vi "QUIZ#1 (interfaz cmd AT).vi"() -> ()   [LabVIEW 2020]
panel:
  out "index of element":i32
  in  "nomtipo":string[](array[string])
  out "element":string
  out "index nombre":i32
  out "before substring":string
  out "es ? , sino sera =":string
  in  "Rpta":string[](array[string])
  in  "Numeric 4":i32
  in  "#args":string[](array[string])
  in  "Numeric 3":i32
  in  "Tipo":string[](array[string])
  in  "Numeric 2":i32
  in  "Nombre":string[](array[string])
  in  "Numeric":i32
  in  "Pulsador 3":bool
  in  "Pulsador 2":bool
  in  "Pulsador 1":bool
  out "Led 3":bool
  out "Led 2":bool
  out "Led 1":bool
  out "tiempo(ms)":i32=2000
  out "Contador":i32
  in  "Insertar trama":string
  out "RESPUESTA":string="\n      \n           "
  in  "Ingreso de comandos":string
  in  "?":bool
  # "DAVID GIRALDO VILLA.\nOSCAR ANDRES CORDOBA."
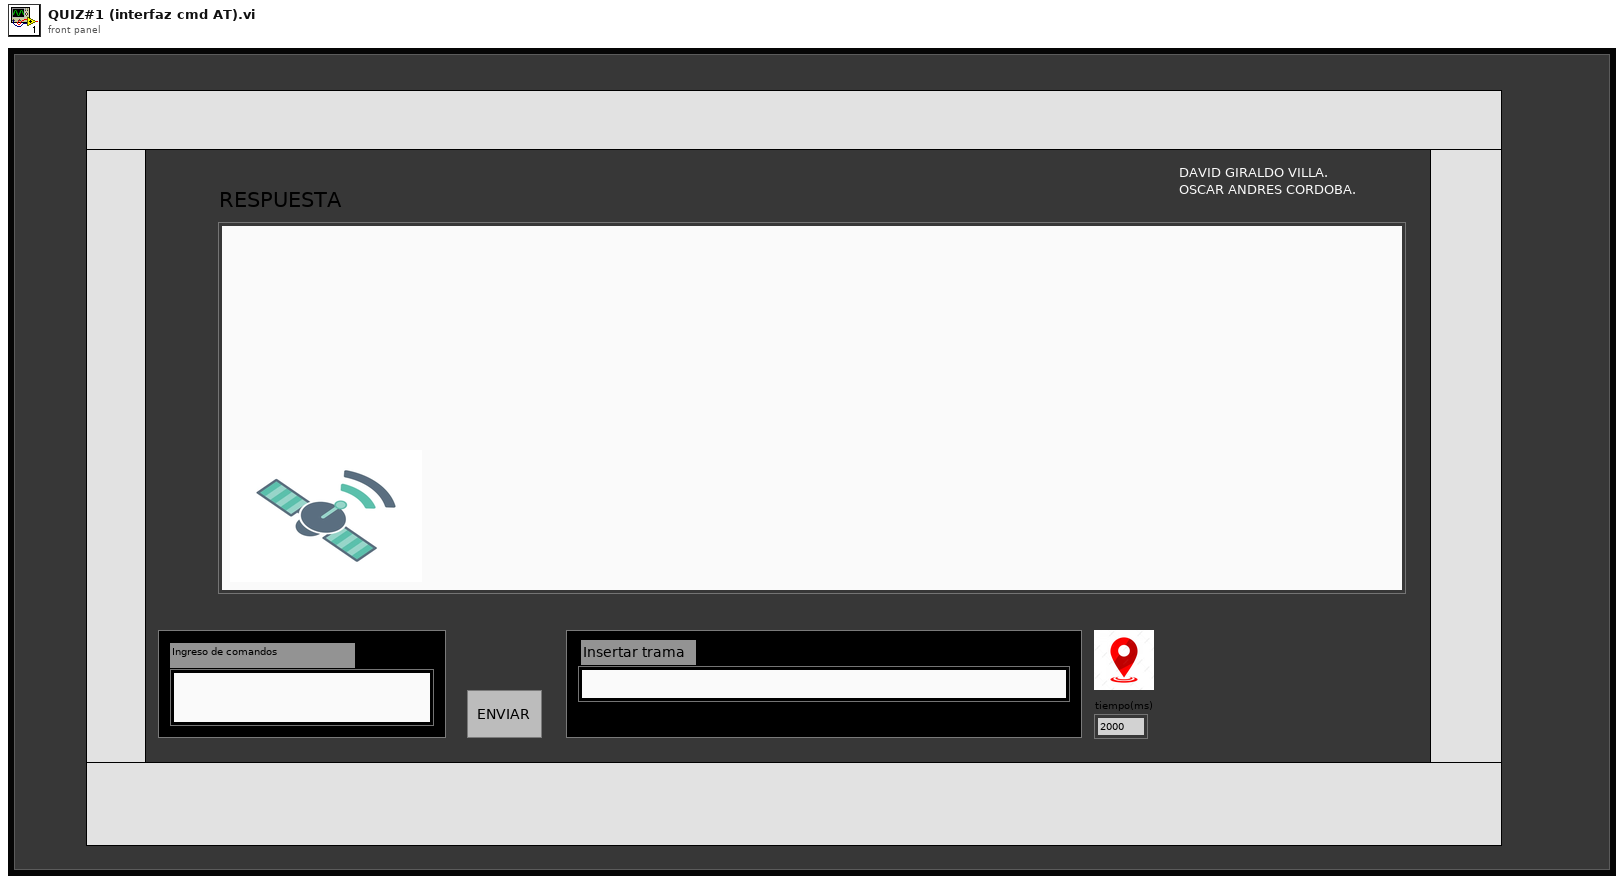
[diagram p1: front panel]
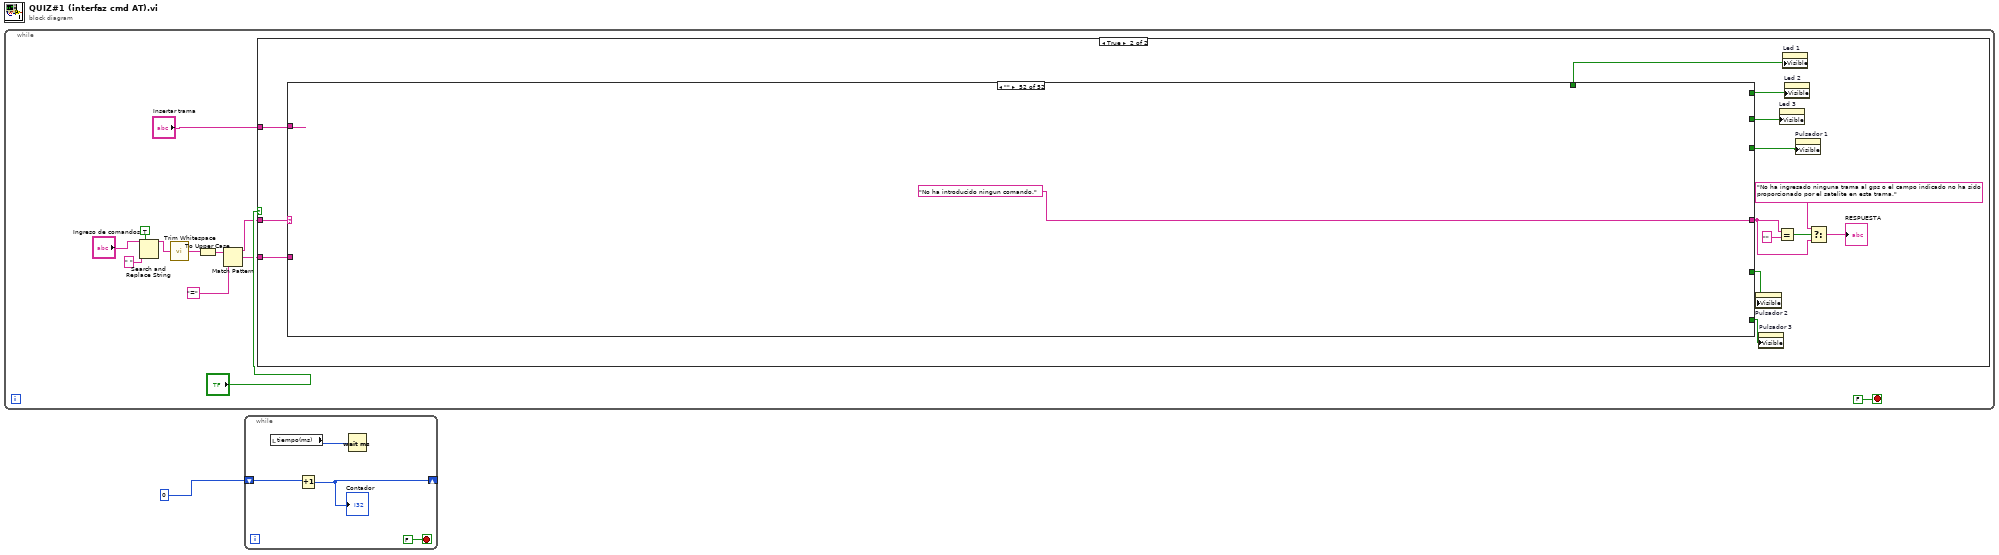
[diagram p0: block diagram]
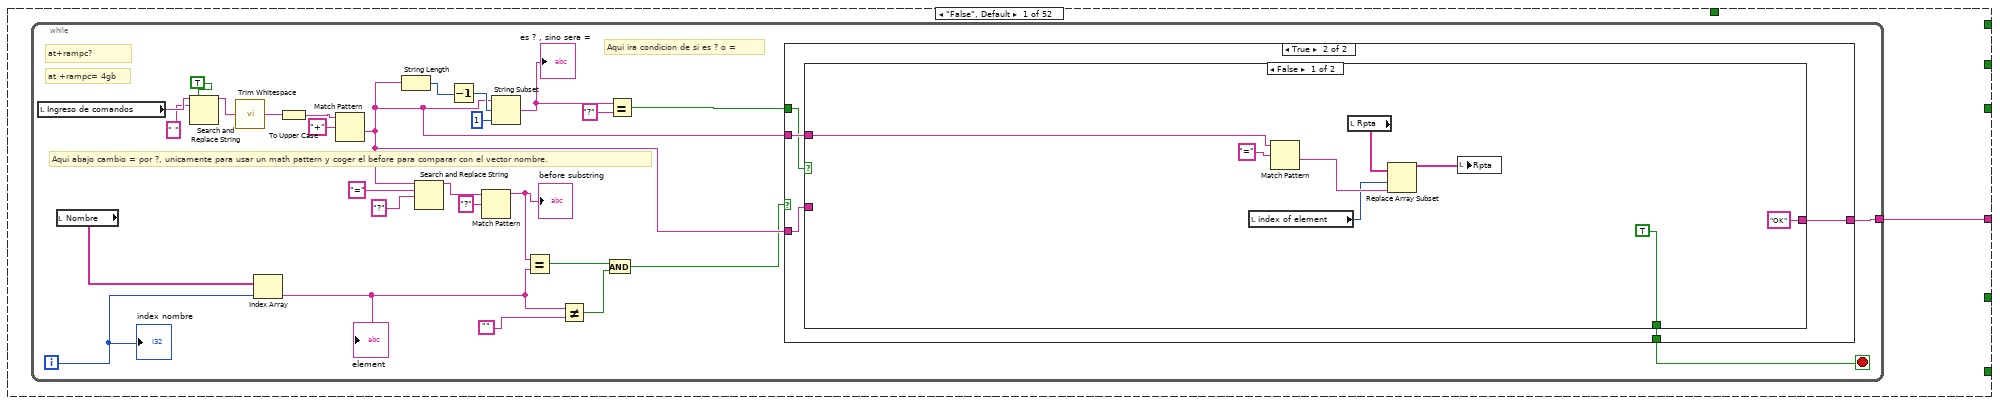
[diagram p3: hidden frame]
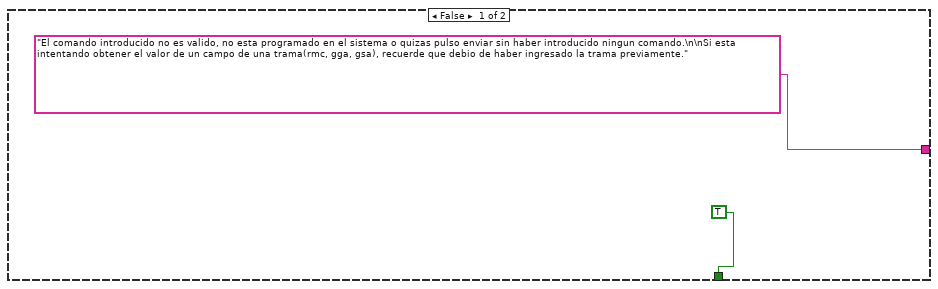
[diagram p4: hidden frame]
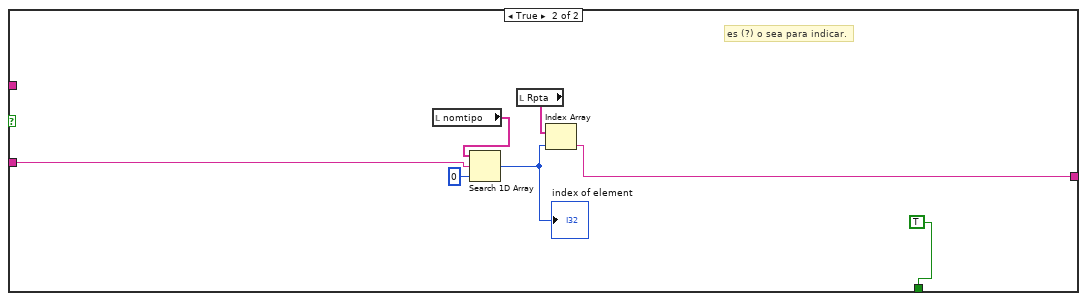
[diagram p5: hidden frame]
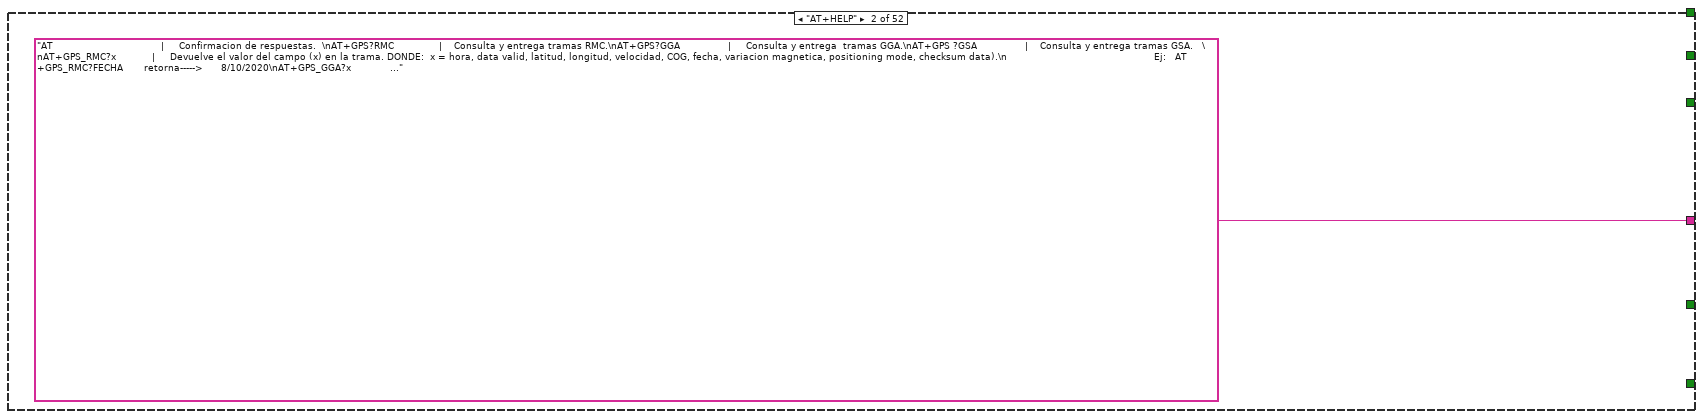
[diagram p6: hidden frame]
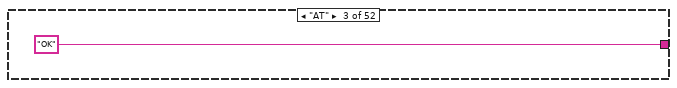
[diagram p7: hidden frame]
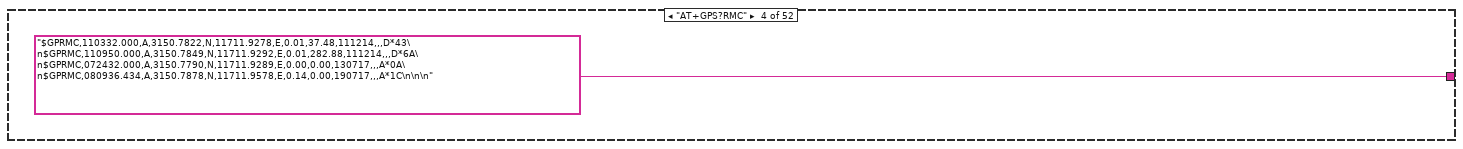
[diagram p8: hidden frame]
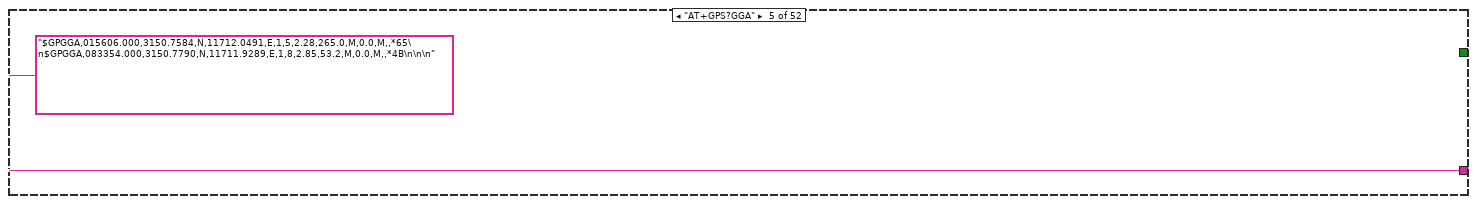
[diagram p9: hidden frame]
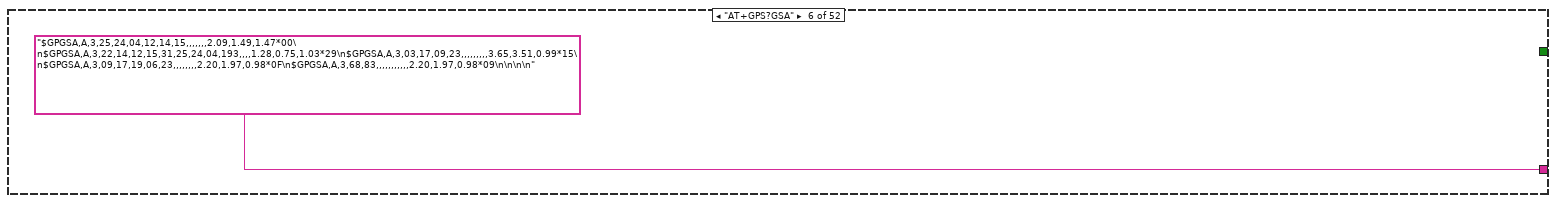
[diagram p10: hidden frame]
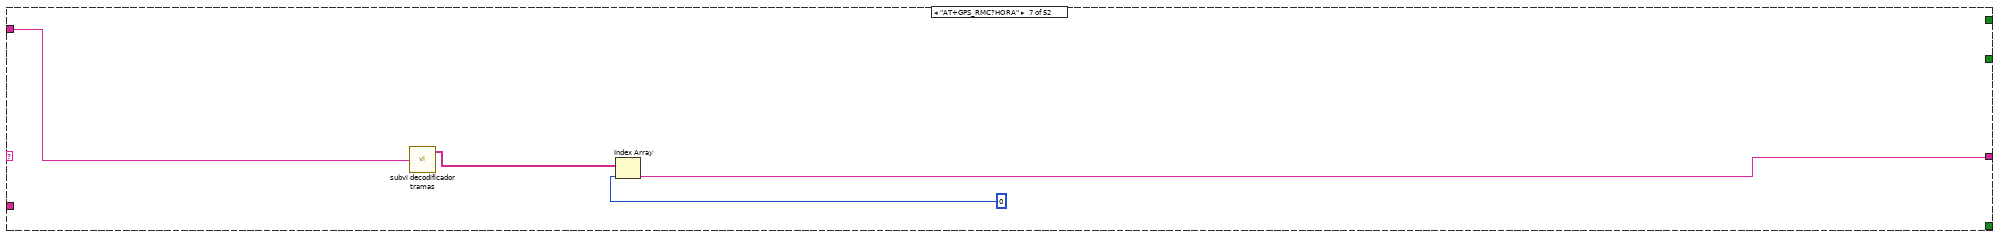
[diagram p11: hidden frame]
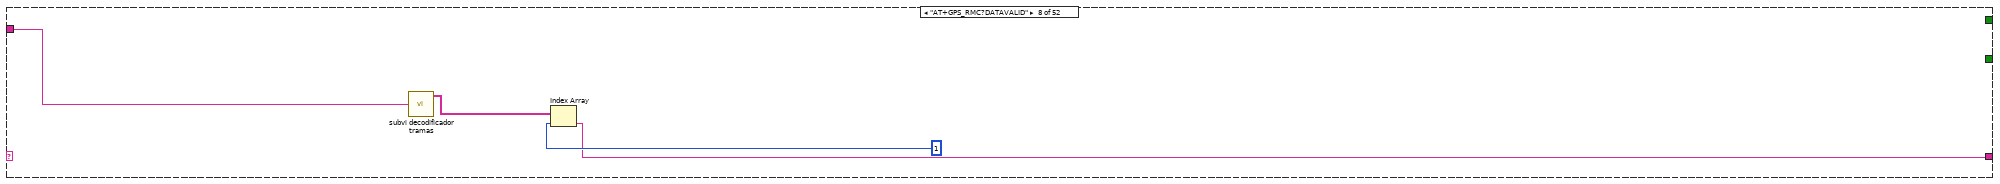
[diagram p12: hidden frame]
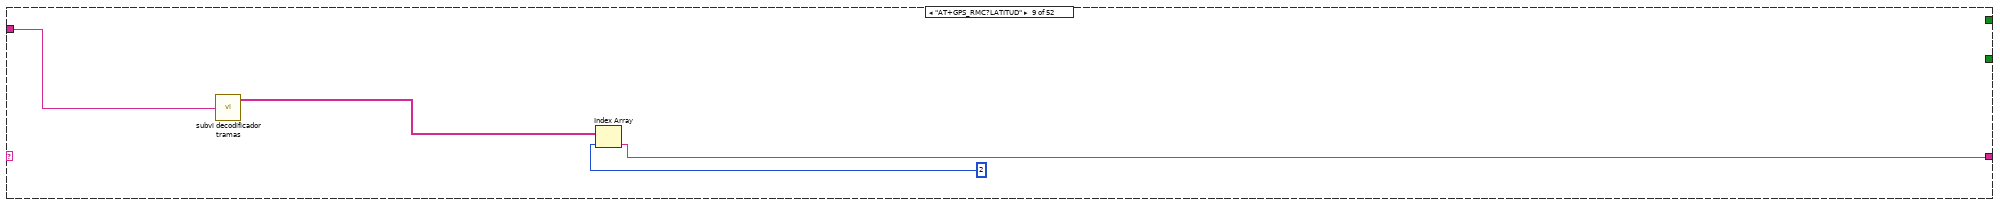
[diagram p13: hidden frame]
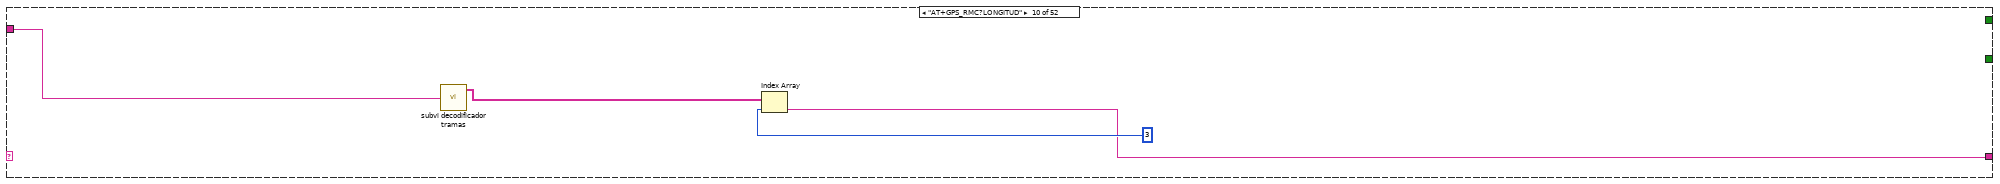
[diagram p14: hidden frame]
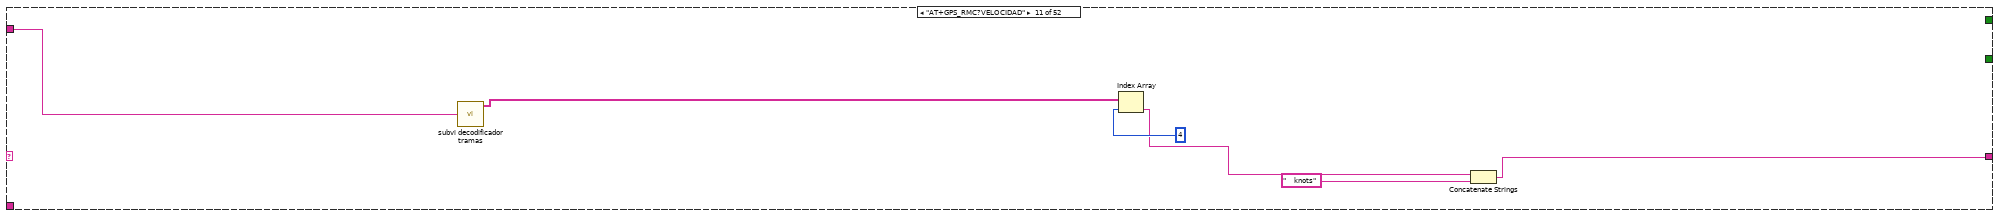
[diagram p15: hidden frame]
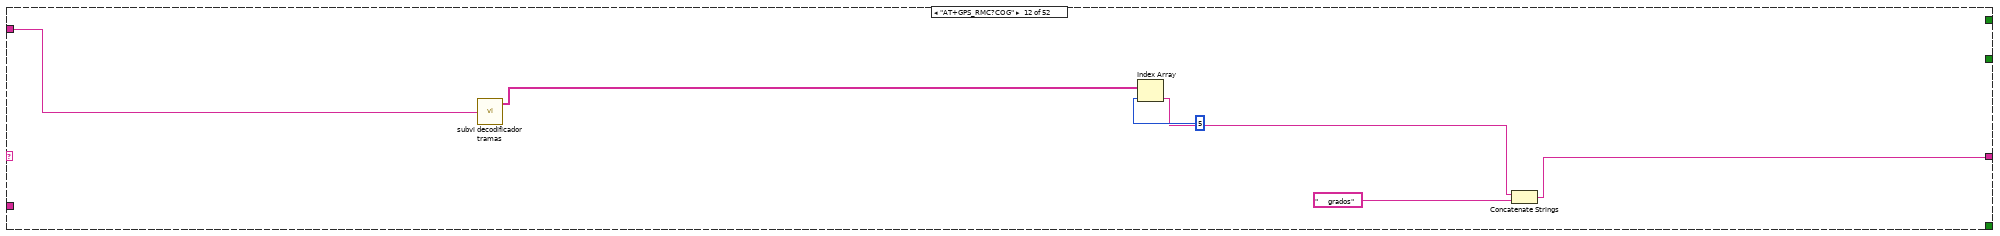
[diagram p16: hidden frame]
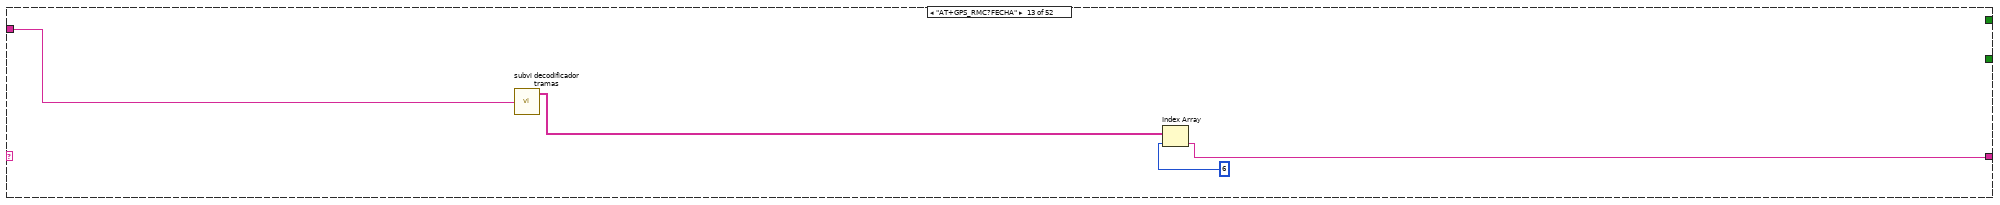
[diagram p17: hidden frame]
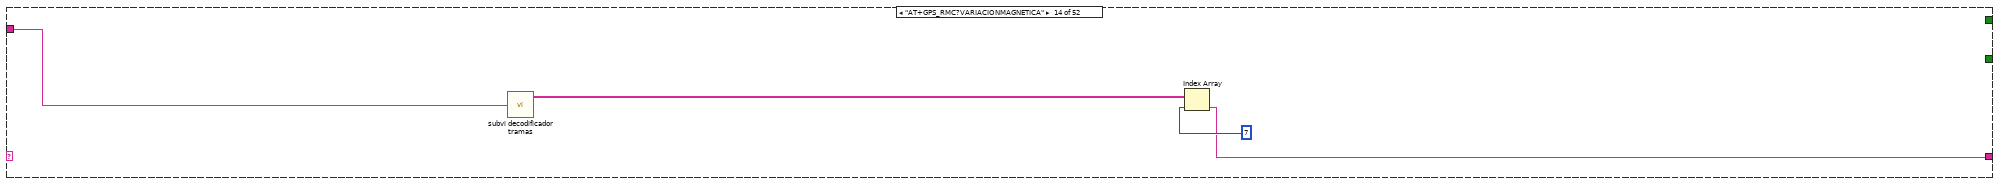
[diagram p18: hidden frame]
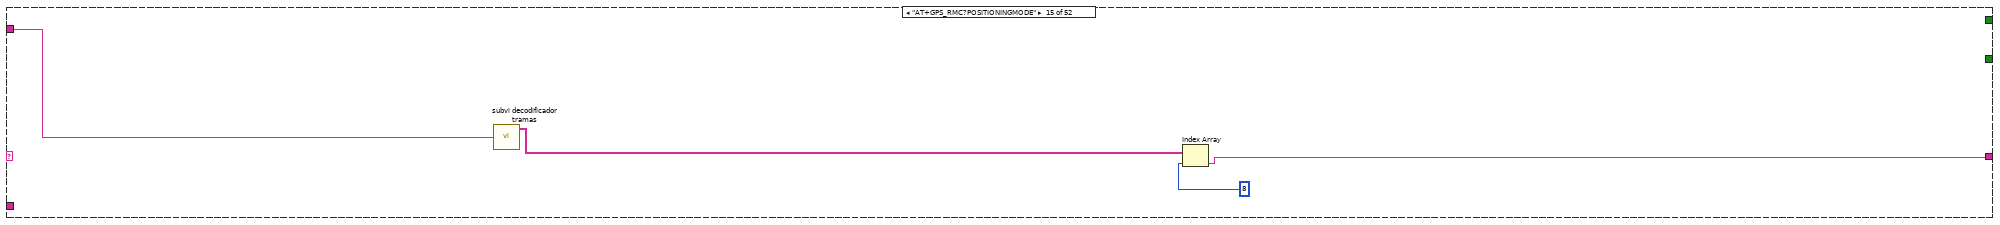
[diagram p19: hidden frame]
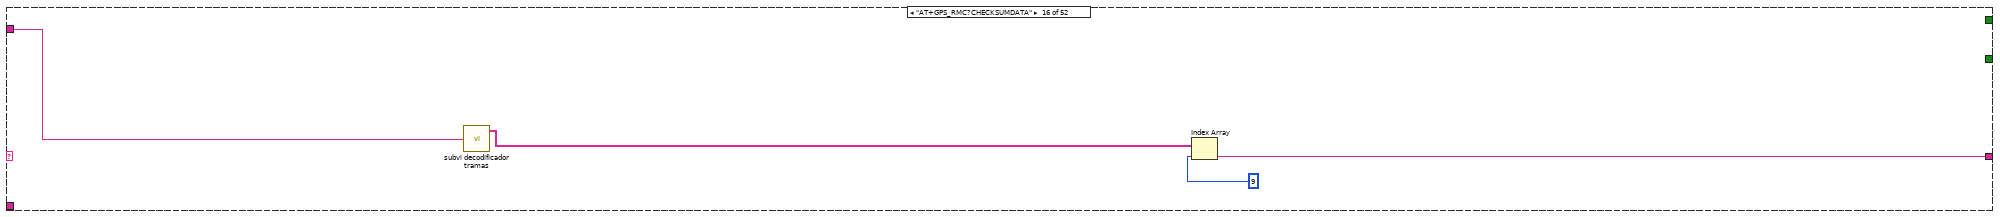
[diagram p20: hidden frame]
diagram:
  n1 = while {
    stop <- FALSE stop-if-true
    n2 = Search and Replace String(replace all?=TRUE ("replace all? (F)"), input string="Ingreso de comandos", search string=" ") -> (result string=w3:string)  [unwired: 5 in, 3 out]
    n3 = call <vilib>:"Trim Whitespace.vi"("string"=w3) -> ("trimmed string"=w2:string)  [unwired: 1 in]
    n4 = To Upper Case(1:w2) -> (0:w12:string)
    n5 = Match Pattern(string=w12, regular expression="=") -> (before substring=w10:string, after substring=w9:string)  [unwired: 1 in, 2 out]
    n6 = case shown="True" "?" {
      tunnel: "Insertar trama" -> [_ w27]
      tunnel: w10 -> [_ w26]
      tunnel: w9 -> [_ w25]
      frame False {
      }
      frame True {
        n7 = case shown="\"\"" w26 {
          tunnel: [w28 "AT                                    |     Confirmacion de respuestas.  \nAT+GPS?RMC               |    Consulta y entrega tramas RMC.\nAT+GPS?GGA                |     Consulta y entrega  tramas GGA.\nAT+GPS ?GSA                |    Consulta y entrega tramas GSA.   \nAT+GPS_RMC?x            |     Devuelve el valor del campo (x) en la trama. DONDE:  x = hora, data valid, latitud, longitud, velocidad, COG, fecha, variacion magnetica, positioning mode, checksum data).\n                                                 Ej:   AT +GPS_RMC?FECHA       retorna----->      8/10/2020\nAT+GPS_GGA?x             |     Devuelve el valor del campo (x) en la trama. DONDE:  x = hora, latitud, longitud, fix status, numero de satelites, HDOP, altitud , Geoid Separation, DGPS AGE, DGPS, ID checksum data).\nAT+GPS_GSA?x              |     Devuelve el valor del campo (x) en la trama. DONDE:  x = mode, fix status, su1, su2, su3, su4, su5, su6, su7, su8 ,su9, su10, su11, su12, PDOP, HDOP, VDOP, checksum data )    y   su: satellite usado.\nAT+TIMEPC                     |     Consulta la hora actual de tu pc.\nAT+CAMBIARTIEMPO=t |  Cambia cada cuanto tiempo aumenta la variable contador.                   DONDE:   t = lapzo de tiempo en (milisegundos) que desea que deba transcurrir para el aumento del contador.\nAT+LEERCONTADOR         | Lee la variable contador.                                                                              \nAT+LEERLEDS                   |  Lee estado de los led.                                                                       \nAT+MODIFICARLEDS      |  Concede a acceso a los pulsadores que envian las señales a los leds para ser modificados.\n\nAT+INSCRIBIR=campo1,campo2,campo3,campo4    ;  Donde: campo1: Nombre del comando a insertar.\n                                                                                                             campo2: Tipo de comando  (Recibir o consultar).\n                                                                                                             campo3: numero de argumentos de argumentos. (que para este programa solo funciona con 1).\n                                                                                                             campo4: Respuesta.\n\n                                                                                      ej:        at+inscribir=rampc,R,1,ok      (comando con tipo recibir o escritura.)        prueba en consola  -->   at+rampc= R\n                                                                                                  at+inscribir=rampc,?,1,4gb     (comando de tipo consulta.)                          prueba en consola -->    at+rampc?\n      \n           " "OK" "$GPRMC,110332.000,A,3150.7822,N,11711.9278,E,0.01,37.48,111214,,,D*43\n$GPRMC,110950.000,A,3150.7849,N,11711.9292,E,0.01,282.88,111214,,,D*6A\n$GPRMC,072432.000,A,3150.7790,N,11711.9289,E,0.00,0.00,130717,,,A*0A\n$GPRMC,080936.434,A,3150.7878,N,11711.9578,E,0.14,0.00,190717,,,A*1C\n\n\n" "$GPGGA,015606.000,3150.7584,N,11712.0491,E,1,5,2.28,265.0,M,0.0,M,,*65\n$GPGGA,083354.000,3150.7790,N,11711.9289,E,1,8,2.85,53.2,M,0.0,M,,*4B\n\n\n" "$GPGSA,A,3,25,24,04,12,14,15,,,,,,,2.09,1.49,1.47*00\n$GPGSA,A,3,22,14,12,15,31,25,24,04,193,,,,1.28,0.75,1.03*29\n$GPGSA,A,3,03,17,09,23,,,,,,,,,3.65,3.51,0.99*15\n$GPGSA,A,3,09,17,19,06,23,,,,,,,,2.20,1.97,0.98*0F\n$GPGSA,A,3,68,83,,,,,,,,,,,2.20,1.97,0.98*09\n\n\n\n" w86 w88 w92 w96 w100 w106 w112 w116 w120 w124 w128 w132 w136 w140 w144 w148 w152 w156 w160 w164 w168 w172 w176 w180 w184 w188 w192 w196 w200 w204 w208 w212 w216 w220 w224 w228 w232 w236 w240 w245 w255 w258 "Los LEDS aparecieron en la parte inferior derecha de la interfaz, dirija su mirada hacia alla para visualizarlos." "Los Pulsadores aparecieron en la parte inferior derecha de la interfaz, dirija su mirada hacia alla para visualizarlos." w272 "No ha introducido ningun comando."] -> w15
          tunnel: w27 -> [_ _ _ _ _ _ w84 w90 w94 w98 w104 w110 w114 w118 w122 w126 w131 w133 w137 w141 w145 w149 w153 w157 w161 w165 w169 w173 w177 w181 w185 w189 w193 w197 w201 w205 w209 w213 w217 w221 w225 w229 w233 w237 w241 _ _ _ _ _ _ _]
          tunnel: [_ _ _ _ _ _ _ _ _ _ _ _ _ _ _ _ _ _ _ _ _ _ _ _ _ _ _ _ _ _ _ _ _ _ _ _ _ _ _ _ _ _ _ _ _ _ _ _ _ w268 _ _] -> w21
          tunnel: [_ _ _ _ _ _ _ _ _ _ _ _ _ _ _ _ _ _ _ _ _ _ _ _ _ _ _ _ _ _ _ _ _ _ _ _ _ _ _ _ _ _ _ _ _ _ _ _ _ w268 _ _] -> w20
          tunnel: [_ _ _ _ _ _ _ _ _ _ _ _ _ _ _ _ _ _ _ _ _ _ _ _ _ _ _ _ _ _ _ _ _ _ _ _ _ _ _ _ _ _ _ _ _ _ _ _ _ w268 _ _] -> w19
          tunnel: w25 -> [_ _ _ _ _ _ _ _ _ _ _ _ _ _ _ _ _ _ _ _ _ _ _ _ _ _ _ _ _ _ _ _ _ _ _ _ _ _ _ _ _ _ _ _ _ _ w257 _ _ _ w277 _]
          tunnel: [_ _ _ _ _ _ _ _ _ _ _ _ _ _ _ _ _ _ _ _ _ _ _ _ _ _ _ _ _ _ _ _ _ _ _ _ _ _ _ _ _ _ _ _ _ _ _ _ w266 _ _ _] -> w24
          tunnel: [_ _ _ _ _ _ _ _ _ _ _ _ _ _ _ _ _ _ _ _ _ _ _ _ _ _ _ _ _ _ _ _ _ _ _ _ _ _ _ _ _ _ _ _ _ _ _ _ w266 _ _ _] -> w23
          tunnel: [_ _ _ _ _ _ _ _ _ _ _ _ _ _ _ _ _ _ _ _ _ _ _ _ _ _ _ _ _ _ _ _ _ _ _ _ _ _ _ _ _ _ _ _ _ _ _ _ w266 _ _ _] -> w22
          frame "False", Default {
            n8 = while {
              tunnel: [w40] -> w28
              i -> [w36]
              stop <- w34 stop-if-true
              # "Aqui abajo cambio = por ?, unicamente para usar un math pattern y coger el before para comparar con el vector nombre."
              # "Aqui ira condicion de si es ? o ="
              # "at+rampc?"
              # "at +rampc= 4gb"
              n9 = local read "Ingreso de comandos"() -> (w55:string)
              n10 = local read "Nombre"() -> (w49:string[])
              n11 = Search and Replace String(replace all?=TRUE ("replace all? (F)"), input string=w55, search string=" ") -> (result string=w53:string)  [unwired: 5 in, 3 out]
              n12 = call <vilib>:"Trim Whitespace.vi"("string"=w53) -> ("trimmed string"=w54:string)  [unwired: 1 in]
              n13 = Index Array(array=w49, index=w36) -> (element=w31:string)
              "element" <- w31
              n14 = To Upper Case(1:w54) -> (0:w56:string)
              n15 = Match Pattern(string=w56, regular expression="+") -> (after substring=w35:string)  [unwired: 1 in, 3 out]
              n16 = String Length(string=w35) -> (length=w48:i32)
              n17 = Search and Replace String(input string=w35, search string="=", replace string="?" ("replace string (\"\")")) -> (result string=w43:string)  [unwired: 5 in, 3 out]
              n18 = Decrement(x=w48) -> (x-1=w47:i32)
              n19 = Match Pattern(string=w43, regular expression="?") -> (before substring=w41:string)  [unwired: 1 in, 3 out]
              "before substring" <- w41
              n20 = String Subset(string=w35, offset (0)=w47, length (rest)=1 ("length (rest)")) -> (substring=w38:string)
              "es ? , sino sera =" <- w38
              n21 = Equal?(x=w41, y=w31) -> (x = y?=w33:bool)
              n22 = Not Equal?(x=w31, y="") -> (x != y?=w30:bool)
              n23 = And(x=w33, y=w30) -> (x .and. y?=w29:bool)
              n24 = Equal?(x=w38, y="?") -> (x = y?=w37:bool)
              n25 = case shown="True" w29 {
                tunnel: ["El comando introducido no es valido, no esta programado en el sistema o quizas pulso enviar sin haber introducido ningun comando.\n\nSi esta intentando obtener el valor de un campo de una trama(rmc, gga, gsa), recuerde que debio de haber ingresado la trama previamente." w62] -> w40
                tunnel: w35 -> [_ w63]
                tunnel: w37 -> [_ w60]
                tunnel: w35 -> [_ w61]
                tunnel: [TRUE w59] -> w34
                frame False {
                }
                frame True {
                  n26 = case shown="False" w60 {
                    tunnel: w63 -> [w70 _]
                    tunnel: ["OK" ("String") w73] -> w62
                    tunnel: w61 -> [_ w74]
                    tunnel: [TRUE TRUE] -> w59
                    frame False {
                      n27 = local read "index of element"() -> (w67:i32)
                      n28 = Match Pattern(string=w70, regular expression="=") -> (after substring=w68:string)  [unwired: 1 in, 3 out]
                      n29 = local read "Rpta"() -> (w69:string[])
                      n30 = Replace Array Subset(array=w69, new element=w68, index=w67) -> (w66:string[])
                      n31 = local write "Rpta"(w66) -> ()
                    }
                    frame True {
                      # "es (?) o sea para indicar."
                      n32 = local read "nomtipo"() -> (w76:string[])
                      n33 = Search 1D Array(1D array=w76, element=w74, start index (0)=0) -> (index of element=w78:i32)
                      "index of element" <- w78
                      n34 = local read "Rpta"() -> (w77:string[])
                      n35 = Index Array(array=w77, index=w78) -> (element=w73:string)
                    }
                  }
                }
              }
              "index nombre" <- w36
            }
          }
          frame "AT+HELP" {
          }
          frame "AT" {
          }
          frame "AT+GPS?RMC" {
          }
          frame "AT+GPS?GGA" {
          }
          frame "AT+GPS?GSA" {
          }
          frame "AT+GPS_RMC?HORA" {
            n36 = call "subvi decodificador tramas.vi"("TRAMA"=w84) -> ("Arreglo salida RMC"=w85:string[])  [unwired: 2 out]
            n37 = Index Array(array=w85, index=0) -> (element=w86:string)
          }
          frame "AT+GPS_RMC?DATAVALID" {
            n38 = call "subvi decodificador tramas.vi"("TRAMA"=w90) -> ("Arreglo salida RMC"=w89:string[])  [unwired: 2 out]
            n39 = Index Array(array=w89, index=1) -> (element=w88:string)
          }
          frame "AT+GPS_RMC?LATITUD" {
            n40 = call "subvi decodificador tramas.vi"("TRAMA"=w94) -> ("Arreglo salida RMC"=w93:string[])  [unwired: 2 out]
            n41 = Index Array(array=w93, index=2) -> (element=w92:string)
          }
          frame "AT+GPS_RMC?LONGITUD" {
            n42 = call "subvi decodificador tramas.vi"("TRAMA"=w98) -> ("Arreglo salida RMC"=w97:string[])  [unwired: 2 out]
            n43 = Index Array(array=w97, index=3) -> (element=w96:string)
          }
          frame "AT+GPS_RMC?VELOCIDAD" {
            n44 = call "subvi decodificador tramas.vi"("TRAMA"=w104) -> ("Arreglo salida RMC"=w103:string[])  [unwired: 2 out]
            n45 = Index Array(array=w103, index=4) -> (element=w101:string)
            n46 = Concatenate Strings(w101, "    knots" ("string")) -> (w100:string)
          }
          frame "AT+GPS_RMC?COG" {
            n47 = call "subvi decodificador tramas.vi"("TRAMA"=w110) -> ("Arreglo salida RMC"=w109:string[])  [unwired: 2 out]
            n48 = Index Array(array=w109, index=5) -> (element=w107:string)
            n49 = Concatenate Strings(w107, "     grados" ("string")) -> (w106:string)
          }
          frame "AT+GPS_RMC?FECHA" {
            n50 = call "subvi decodificador tramas.vi"("TRAMA"=w114) -> ("Arreglo salida RMC"=w113:string[])  [unwired: 2 out]
            n51 = Index Array(array=w113, index=6) -> (element=w112:string)
          }
          frame "AT+GPS_RMC?VARIACIONMAGNETICA" {
            n52 = call "subvi decodificador tramas.vi"("TRAMA"=w118) -> ("Arreglo salida RMC"=w117:string[])  [unwired: 2 out]
            n53 = Index Array(array=w117, index=7) -> (element=w116:string)
          }
          frame "AT+GPS_RMC?POSITIONINGMODE" {
            n54 = call "subvi decodificador tramas.vi"("TRAMA"=w122) -> ("Arreglo salida RMC"=w121:string[])  [unwired: 2 out]
            n55 = Index Array(array=w121, index=8) -> (element=w120:string)
          }
          frame "AT+GPS_RMC?CHECKSUMDATA" {
            n56 = call "subvi decodificador tramas.vi"("TRAMA"=w126) -> ("Arreglo salida RMC"=w125:string[])  [unwired: 2 out]
            n57 = Index Array(array=w125, index=9) -> (element=w124:string)
          }
          frame "AT+GPS_GGA?HORA" {
            n58 = call "subvi decodificador tramas.vi"("TRAMA"=w131) -> ("Arreglo salida GGA"=w129:string[])  [unwired: 2 out]
            n59 = Index Array(array=w129, index=0) -> (element=w128:string)
          }
          frame "AT+GPS_GGA?LATITUD" {
            n60 = call "subvi decodificador tramas.vi"("TRAMA"=w133) -> ("Arreglo salida GGA"=w134:string[])  [unwired: 2 out]
            n61 = Index Array(array=w134, index=1) -> (element=w132:string)
          }
          frame "AT+GPS_GGA?LONGITUD" {
            n62 = call "subvi decodificador tramas.vi"("TRAMA"=w137) -> ("Arreglo salida GGA"=w138:string[])  [unwired: 2 out]
            n63 = Index Array(array=w138, index=2) -> (element=w136:string)
          }
          frame "AT+GPS_GGA?FIXSTATUS" {
            n64 = call "subvi decodificador tramas.vi"("TRAMA"=w141) -> ("Arreglo salida GGA"=w142:string[])  [unwired: 2 out]
            n65 = Index Array(array=w142, index=3) -> (element=w140:string)
          }
          frame "AT+GPS_GGA?NUMERODESATELITES" {
            n66 = call "subvi decodificador tramas.vi"("TRAMA"=w145) -> ("Arreglo salida GGA"=w146:string[])  [unwired: 2 out]
            n67 = Index Array(array=w146, index=4) -> (element=w144:string)
          }
          frame "AT+GPS_GGA?HDOP" {
            n68 = call "subvi decodificador tramas.vi"("TRAMA"=w149) -> ("Arreglo salida GGA"=w150:string[])  [unwired: 2 out]
            n69 = Index Array(array=w150, index=5) -> (element=w148:string)
          }
          frame "AT+GPS_GGA?ALTITUD" {
            n70 = call "subvi decodificador tramas.vi"("TRAMA"=w153) -> ("Arreglo salida GGA"=w154:string[])  [unwired: 2 out]
            n71 = Index Array(array=w154, index=6) -> (element=w152:string)
          }
          frame "AT+GPS_GGA?GEOIDSEPARATION" {
            n72 = call "subvi decodificador tramas.vi"("TRAMA"=w157) -> ("Arreglo salida GGA"=w158:string[])  [unwired: 2 out]
            n73 = Index Array(array=w158, index=7) -> (element=w156:string)
          }
          frame "AT+GPS_GGA?DGPSAGE" {
            n74 = call "subvi decodificador tramas.vi"("TRAMA"=w161) -> ("Arreglo salida GGA"=w162:string[])  [unwired: 2 out]
            n75 = Index Array(array=w162, index=8) -> (element=w160:string)
          }
          frame "AT+GPS_GGA?DGPSID" {
            n76 = call "subvi decodificador tramas.vi"("TRAMA"=w165) -> ("Arreglo salida GGA"=w166:string[])  [unwired: 2 out]
            n77 = Index Array(array=w166, index=9) -> (element=w164:string)
          }
          frame "AT+GPS_GGA?CHECKSUMDATA" {
            n78 = call "subvi decodificador tramas.vi"("TRAMA"=w169) -> ("Arreglo salida GGA"=w170:string[])  [unwired: 2 out]
            n79 = Index Array(array=w170, index=10) -> (element=w168:string)
          }
          frame "AT+GPS_GSA?MODE" {
            n80 = call "subvi decodificador tramas.vi"("TRAMA"=w173) -> ("Arreglo salida GSA"=w174:string[])  [unwired: 2 out]
            n81 = Index Array(array=w174, index=0) -> (element=w172:string)
          }
          frame "AT+GPS_GSA?FIXSTATUS" {
            n82 = call "subvi decodificador tramas.vi"("TRAMA"=w177) -> ("Arreglo salida GSA"=w178:string[])  [unwired: 2 out]
            n83 = Index Array(array=w178, index=1) -> (element=w176:string)
          }
          frame "AT+GPS_GSA?SU1" {
            n84 = call "subvi decodificador tramas.vi"("TRAMA"=w181) -> ("Arreglo salida GSA"=w182:string[])  [unwired: 2 out]
            n85 = Index Array(array=w182, index=2) -> (element=w180:string)
          }
          frame "AT+GPS_GSA?SU2" {
            n86 = call "subvi decodificador tramas.vi"("TRAMA"=w185) -> ("Arreglo salida GSA"=w186:string[])  [unwired: 2 out]
            n87 = Index Array(array=w186, index=3) -> (element=w184:string)
          }
          frame "AT+GPS_GSA?SU3" {
            n88 = call "subvi decodificador tramas.vi"("TRAMA"=w189) -> ("Arreglo salida GSA"=w190:string[])  [unwired: 2 out]
            n89 = Index Array(array=w190, index=4) -> (element=w188:string)
          }
          frame "AT+GPS_GSA?SU4" {
            n90 = call "subvi decodificador tramas.vi"("TRAMA"=w193) -> ("Arreglo salida GSA"=w194:string[])  [unwired: 2 out]
            n91 = Index Array(array=w194, index=5) -> (element=w192:string)
          }
          frame "AT+GPS_GSA?SU5" {
            n92 = call "subvi decodificador tramas.vi"("TRAMA"=w197) -> ("Arreglo salida GSA"=w198:string[])  [unwired: 2 out]
            n93 = Index Array(array=w198, index=6) -> (element=w196:string)
          }
          frame "AT+GPS_GSA?SU6" {
            n94 = call "subvi decodificador tramas.vi"("TRAMA"=w201) -> ("Arreglo salida GSA"=w202:string[])  [unwired: 2 out]
            n95 = Index Array(array=w202, index=7) -> (element=w200:string)
          }
          frame "AT+GPS_GSA?SU7" {
            n96 = call "subvi decodificador tramas.vi"("TRAMA"=w205) -> ("Arreglo salida GSA"=w206:string[])  [unwired: 2 out]
            n97 = Index Array(array=w206, index=8) -> (element=w204:string)
          }
          frame "AT+GPS_GSA?SU8" {
            n98 = call "subvi decodificador tramas.vi"("TRAMA"=w209) -> ("Arreglo salida GSA"=w210:string[])  [unwired: 2 out]
            n99 = Index Array(array=w210, index=9) -> (element=w208:string)
          }
          frame "AT+GPS_GSA?SU9" {
            n100 = call "subvi decodificador tramas.vi"("TRAMA"=w213) -> ("Arreglo salida GSA"=w214:string[])  [unwired: 2 out]
            n101 = Index Array(array=w214, index=10) -> (element=w212:string)
          }
          frame "AT+GPS_GSA?SU10" {
            n102 = call "subvi decodificador tramas.vi"("TRAMA"=w217) -> ("Arreglo salida GSA"=w218:string[])  [unwired: 2 out]
            n103 = Index Array(array=w218, index=11) -> (element=w216:string)
          }
          frame "AT+GPS_GSA?SU11" {
            n104 = call "subvi decodificador tramas.vi"("TRAMA"=w221) -> ("Arreglo salida GSA"=w222:string[])  [unwired: 2 out]
            n105 = Index Array(array=w222, index=12) -> (element=w220:string)
          }
          frame "AT+GPS_GSA?SU12" {
            n106 = call "subvi decodificador tramas.vi"("TRAMA"=w225) -> ("Arreglo salida GSA"=w226:string[])  [unwired: 2 out]
            n107 = Index Array(array=w226, index=13) -> (element=w224:string)
          }
          frame "AT+GPS_GSA?PDOP" {
            n108 = call "subvi decodificador tramas.vi"("TRAMA"=w229) -> ("Arreglo salida GSA"=w230:string[])  [unwired: 2 out]
            n109 = Index Array(array=w230, index=14) -> (element=w228:string)
          }
          frame "AT+GPS_GSA?HDOP" {
            n110 = call "subvi decodificador tramas.vi"("TRAMA"=w233) -> ("Arreglo salida GSA"=w234:string[])  [unwired: 2 out]
            n111 = Index Array(array=w234, index=15) -> (element=w232:string)
          }
          frame "AT+GPS_GSA?VDOP" {
            n112 = call "subvi decodificador tramas.vi"("TRAMA"=w237) -> ("Arreglo salida GSA"=w238:string[])  [unwired: 2 out]
            n113 = Index Array(array=w238, index=16) -> (element=w236:string)
          }
          frame "AT+GPS_GSA?CHECKSUMDATA" {
            n114 = call "subvi decodificador tramas.vi"("TRAMA"=w241) -> ("Arreglo salida GSA"=w242:string[])  [unwired: 2 out]
            n115 = Index Array(array=w242, index=17) -> (element=w240:string)
          }
          frame "AT+TIMEPC" {
            n116 = Get Date/Time String() -> (date string=w250:string, time string=w248:string)  [unwired: 3 in]
            n117 = Concatenate Strings("Fecha: " ("string"), w250) -> (w247:string)
            n118 = Concatenate Strings("Hora: " ("string"), w248) -> (w246:string)
            n119 = Concatenate Strings(w247, "\r\n", w246) -> (w245:string)
          }
          frame "AT+CAMBIARTIEMPO" {
            n120 = Decimal String To Number(string=w257) -> (number=w256:i32)  [unwired: 2 in, 1 out]
            "tiempo(ms)" <- w256
            n121 = Number To Decimal String(number=w256) -> (decimal integer string=w253:string)  [unwired: 1 in]
            n122 = Concatenate Strings("El tiempo ha sido modificado. visualice en el indicador de abajo llamado tiempo(ms).\n\nEl nuevo tiempo indicado es:       ", w253, "    milisegundos") -> (w255:string)
          }
          frame "AT+LEERCONTADOR" {
            n123 = local read "Contador"() -> (w261:i32)
            n124 = Number To Decimal String(number=w261) -> (decimal integer string=w259:string)  [unwired: 1 in]
            n125 = Concatenate Strings("El valor actual del contador es:    " ("string"), w259) -> (w258:string)
          }
          frame "AT+LEERLEDS" {
            w266 = TRUE
            n126 = local read "Pulsador 2"() -> (→"Led 2":bool)
            n127 = local read "Pulsador 1"() -> (→"Led 1":bool)
            n128 = local read "Pulsador 3"() -> (→"Led 3":bool)
          }
          frame "AT+MODIFICARLEDS" {
            w268 = TRUE
          }
          frame "AT+INSCRIBIR" {
            n129 = Search and Replace String(replace all?=TRUE ("replace all? (F)"), input string=w277, search string=",", replace string="," ("replace string (\"\")")) -> (result string=w273:string, number of replacements=w270:i32)  [unwired: 4 in, 2 out]
            n130 = Equal?(x=3, y=w270) -> (x = y?=w269:bool)
            n131 = case shown="True" w269 {
              tunnel: w273 -> [_ w281]
              tunnel: ["El comando inscrito esta incorrecto, recuerde que debe de tener 4 parametros:\n\nat+insertar=nombre,tipo,#args,respuesta" "Inscribiendo comando..."] -> w272
              tunnel: w270 -> [_ w279]
              frame False {
              }
              frame True {
                n132 = for {
                  N: w279 -> [_]
                  shift-right: [w283] -> _
                  shift-left: w281 -> [w284]
                  i -> [w282]
                  n133 = Match Pattern(string=w284, regular expression=",") -> (before substring=w285:string, after substring=w283:string)  [unwired: 1 in, 2 out]
                  n134 = case shown="2" w282 {
                    tunnel: w285 -> [_ w287 w297 w318]
                    tunnel: w283 -> [_ _ _ w315]
                    tunnel: w282 -> [_ _ _ _]
                    frame 5, Default {
                    }
                    frame 0 {
                      n135 = flat-sequence {
                        tunnel: ["Numeric"] -> w289
                        tunnel: [w291] -> w288
                        tunnel: w289 -> [w291]
                        tunnel: w287 -> [w293]
                        tunnel: ["Nombre"] -> _
                        tunnel: [w291] -> _
                        tunnel: w288 -> [w295]
                        frame #0 {
                        }
                        frame #1 {
                          n136 = Insert Into Array(array="Nombre", index=w291, new element=w293) -> (w294:string[])
                          n137 = property on="Nombre" class="Arr (strict)"("Value"=w294) -> ()  [unwired: 2 in, 2 out]
                        }
                        frame #2 {
                          n138 = Increment(x=w295) -> (x+1=w296:i32)
                          n139 = local write "Numeric"(w296) -> ()
                        }
                      }
                    }
                    frame 1 {
                      n140 = flat-sequence {
                        tunnel: ["Numeric 2"] -> w299
                        tunnel: [w302] -> w298
                        tunnel: w299 -> [w302]
                        tunnel: w297 -> [w303]
                        tunnel: [w302] -> _
                        tunnel: ["Tipo"] -> _
                        tunnel: w298 -> [w305]
                        frame #0 {
                        }
                        frame #1 {
                          n141 = Insert Into Array(array="Tipo", index=w302, new element=w303) -> (w304:string[])
                          n142 = property on="Tipo" class="Arr (strict)"("Value"=w304) -> ()  [unwired: 2 in, 2 out]
                        }
                        frame #2 {
                          n143 = Increment(x=w305) -> (x+1=w306:i32)
                          n144 = local write "Numeric 2"(w306) -> ()
                        }
                      }
                    }
                    frame 2 {
                      n145 = flat-sequence {
                        tunnel: ["Numeric 3"] -> w320
                        tunnel: [w332] -> w319
                        tunnel: w320 -> [w332]
                        tunnel: w318 -> [_]
                        tunnel: w319 -> [w333]
                        frame #0 {
                        }
                        frame #1 {
                          n146 = Insert Into Array(array="#args", index=w332, new element="1") -> (w330:string[])
                          n147 = property on="#args" class="Arr (strict)"("Value"=w330) -> ()  [unwired: 2 in, 2 out]
                        }
                        frame #2 {
                          n148 = Increment(x=w333) -> (x+1=w334:i32)
                          n149 = local write "Numeric 3"(w334) -> ()
                        }
                      }
                      n150 = flat-sequence {
                        tunnel: ["Numeric 4"] -> w317
                        tunnel: [w322] -> w316
                        tunnel: w317 -> [w322]
                        tunnel: w315 -> [w323]
                        tunnel: [w322] -> w307
                        tunnel: w316 -> [w326]
                        frame #0 {
                        }
                        frame #1 {
                          n151 = Insert Into Array(array="Rpta", index=w322, new element=w323) -> (w324:string[])
                          n152 = property on="Rpta" class="Arr (strict)"("Value"=w324) -> ()  [unwired: 2 in, 2 out]
                        }
                        frame #2 {
                          n153 = Increment(x=w326) -> (x+1=w327:i32)
                          n154 = local write "Numeric 4"(w327) -> ()
                        }
                      }
                      n155 = local read "Tipo"() -> (w309:string[])
                      n156 = local read "Nombre"() -> (w311:string[])
                      n157 = Index Array(array=w311, index=w307) -> (element=w310:string)
                      n158 = Index Array(array=w309, index=w307) -> (element=w308:string)
                      n159 = Concatenate Strings(w310, w308) -> (w313:string)
                      n160 = Insert Into Array(array="nomtipo", new element=w313) -> (w314:string[])  [unwired: 1 in]
                      n161 = property on="nomtipo" class="Arr (strict)"("Value"=w314) -> ()  [unwired: 2 in, 2 out]
                    }
                  }
                }
              }
            }
          }
          frame "" {
          }
        }
        n162 = property on="Pulsador 2" class="Bool (strict)"("Visible"=w20) -> ()  [unwired: 2 in, 2 out]
        n163 = property on="Pulsador 3" class="Bool (strict)"("Visible"=w19) -> ()  [unwired: 2 in, 2 out]
        n164 = Equal?(x=w15, y="") -> (x = y?=w17:bool)
        n165 = property on="Led 3" class="Bool (strict)"("Visible"=w22) -> ()  [unwired: 2 in, 2 out]
        n166 = property on="Led 1" class="Bool (strict)"("Visible"=w24) -> ()  [unwired: 2 in, 2 out]
        n167 = property on="Led 2" class="Bool (strict)"("Visible"=w23) -> ()  [unwired: 2 in, 2 out]
        n168 = property on="Pulsador 1" class="Bool (strict)"("Visible"=w21) -> ()  [unwired: 2 in, 2 out]
        n169 = Select(t="No ha ingresado ninguna trama al gps o el campo indicado no ha sido proporcionado por el satelite en esta trama." ("y"), s=w17, f=w15) -> (s? t:f=→"RESPUESTA":string)
      }
    }
  }
  n170 = while {
    shift-right: [w336] -> _
    shift-left: 0 -> [w339]
    stop <- FALSE stop-if-true
    n171 = local read "tiempo(ms)"() -> (w337:i32)
    n172 = Increment(x=w339) -> (x+1=w336:i32)
    "Contador" <- w336
    n173 = Wait (ms)(milliseconds to wait=w337) -> ()  [unwired: 1 out]
  }
